vi "Set Session Handle Queue.vi"(0 "OBJ - Session in":refnum<class "niRFUtil Session.lvclass">, 5 "Session Queue Handle":refnum<queue>, 11 "error in (no error)":errorcluster) -> (4 "OBJ - Session out":refnum<class "niRFUtil Session.lvclass">, 6 "Stored new reference":bool, 15 "error out":errorcluster)   [LabVIEW 2016, in "niRFUtil.lvlib" / "niRFUtil Session.lvclass"]
doc: "Pass the notifier reference into the class.\n\nNotifier reference is stored so that it's possilbe to release the reference on session close."
uses:
  niRFUtil Session.lvclass
  niRFUtil Session.lvclass/niRFUtil Session.ctl
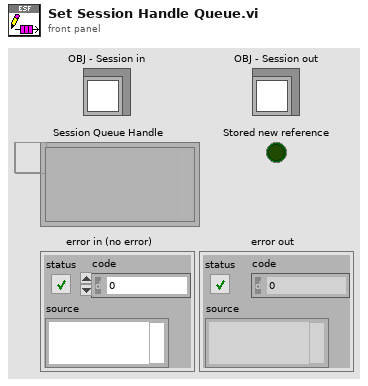
[diagram p1: front panel]
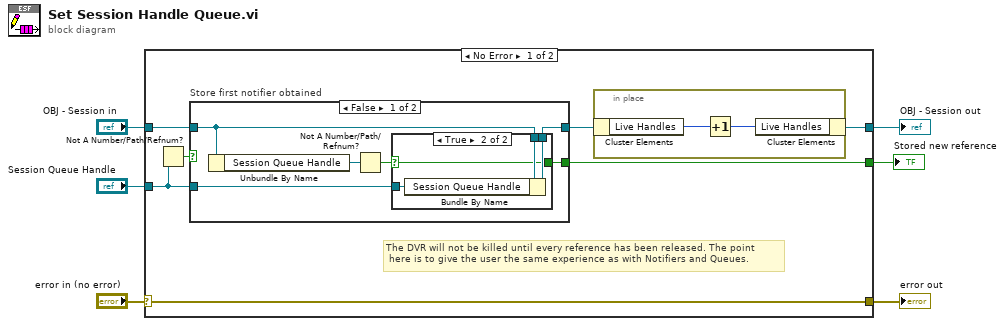
[diagram p0: block diagram]
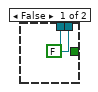
[diagram p2: hidden frame]
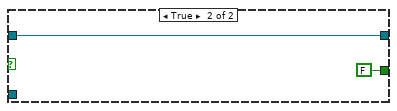
[diagram p3: hidden frame]
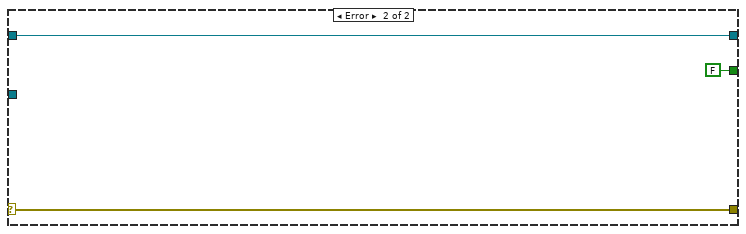
[diagram p4: hidden frame]
diagram:
  n1 = case shown="No Error" "error in (no error)" {
    selector: "error in (no error)" -> [w13 w31]
    tunnel: [w13 w31] -> w5
    tunnel: [w10 w32] -> w3
    tunnel: "OBJ - Session in" -> [w12 w32]
    tunnel: "Session Queue Handle" -> [w9 _]
    tunnel: [w7 FALSE] -> w1
    frame No Error {
      # "The DVR will not be killed until every reference has been released. The point\n here is to give the user the same experience as with Notifiers and Queues."
      n2 = Not A Number/Path/Refnum?(number/path/refnum=w9) -> (NaN/Path/Refnum?=w8:bool)
      n3 = case "Store first notifier obtained" shown="False" w8 {
        tunnel: w12 -> [w15 w27]
        tunnel: w9 -> [w19 _]
        tunnel: [w18 w27] -> w11
        tunnel: [w14 FALSE] -> w7
        frame False {
          n4 = Unbundle By Name(w15) -> ("Session Queue Handle"=w17:refnum<queue>)
          n5 = Not A Number/Path/Refnum?(number/path/refnum=w17) -> (NaN/Path/Refnum?=w16:bool)
          n6 = case shown="True" w16 {
            selector: w16 -> [_ w22]
            tunnel: w19 -> [_ w25]
            tunnel: [w21 w24] -> w18
            tunnel: w15 -> [w21 w23]
            tunnel: [FALSE w22] -> w14
            frame False {
            }
            frame True {
              n7 = Bundle By Name(cluster=w23, "Session Queue Handle"=w25) -> (w24:refnum<class "niRFUtil Session.lvclass">)
            }
          }
        }
        frame True {
        }
      }
      n8 = in-place {
        n9 = in-place-cluster #1(w11) -> ("Live Handles"=w29:u32)
        n10 = Increment(x=w29) -> (x+1=w28:u32)
        n11 = in-place-cluster #1("Live Handles"=w28) -> (w10:refnum<class "niRFUtil Session.lvclass">)
      }
    }
    frame Error {
    }
  }
  "error out" <- w5
  "OBJ - Session out" <- w3
  "Stored new reference" <- w1
